vi "Get Client Certificates (Server).vi"(10 "Client Certificates":T1) -> (2 "trusted client certificates":path[](array[path]))   [LabVIEW 2013, in "OPC UA Client Tests.lvlib"]
doc: "Build paths to server's trusted client certificates."
uses:
  OPC UA Client Tests.lvlib
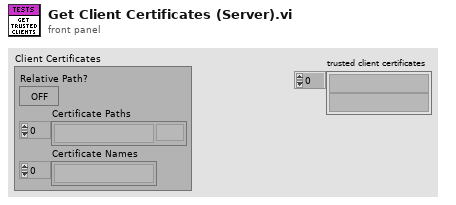
[diagram p1: front panel]
types:
  T1 = cluster{"Relative Path?":bool, "Certificate Paths":path[], "Certificate Names":string[]}
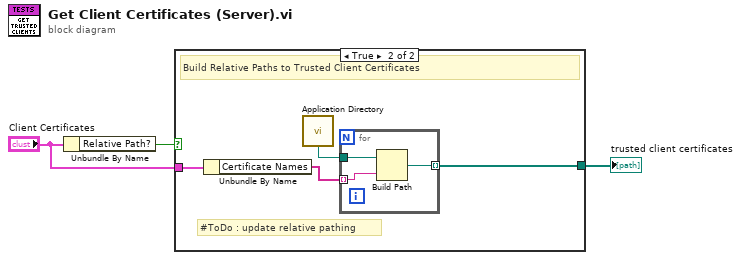
[diagram p0: block diagram]
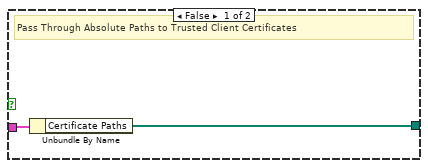
[diagram p2: hidden frame]
diagram:
  n1 = Unbundle By Name("Client Certificates") -> ("Relative Path?"=w3:bool)
  n2 = case shown="True" w3 {
    tunnel: "Client Certificates" -> [w5 w9]
    tunnel: [w4 w6] -> w1
    frame False {
      # "Pass Through Absolute Paths to Trusted Client Certificates"
      n3 = Unbundle By Name(w5) -> ("Certificate Paths"=w4:path[])
    }
    frame True {
      # "#ToDo : update relative pathing"
      # "Build Relative Paths to Trusted Client Certificates"
      n4 = Unbundle By Name(w9) -> ("Certificate Names"=w8:string[])
      n5 = call <vilib>:"Application Directory.vi"() -> ("Application Directory"=w7:path)
      n6 = for {
        tunnel: w8 -> [w11] mode=indexing
        tunnel: w7 -> [w12]
        tunnel: [w10] -> w6 mode=indexing
        n7 = Build Path(base path=w12, name or relative path=w11) -> (appended path=w10:path)
      }
    }
  }
  "trusted client certificates" <- w1
